vi "OAT Unfiltered Orbit Plot (Resampled).vi"(0 "resampled signal(X)":cluster{"r0":dbl, "dr":dbl, "Y":dbl[]} {"r0" format="%.2p"; "dr" format="%.2p"; "Y" format="%.2f"}, 1 "XY graph Ref":refnum<vi>, 5 "resampled signal (Y)":cluster{"r0":dbl, "dr":dbl, "Y":dbl[]} {"r0" format="%.2p"; "dr" format="%.2p"; "Y" format="%.2f"}, 7 "speed profile":T1 {"speed [RPM]" format="%.2f"; "time [s]" format="%.2f"}, 9 "pulse/revolution (1)":i32=1, 11 "error in (no error)":errorcluster, 12 "orbit segment":cluster{"position":dbl, "tach duty":dbl}={"position"=0.0, "tach duty"=0.98} {"tach duty" format="%.2f"; "position" format="%.2f"}, 13 "probe angle":u16(ring) items=["0", "45", "90", "135", "180", "225", "270", "315"]) -> (4 "XY plot value":cluster{"X":dbl[], "Y":dbl[]}[](array[cluster]) {"Y" format="%.2f"; "X" format="%.2f"}, 15 "error out":errorcluster)   [LabVIEW 2017]
doc: "Draws an orbit plot of waveform signals on a XY graph. You can use sampled or resampled waveform signals from proximity transducers. You can use this polymorphic VI to draw an orbit plot of resampled signals or waveform signals. The data types you wire to the <B>resampled signal(X)</B> and <B>resampled signal (Y)</B> inputs determine the polymorphic instance to use."
uses:
  <vilib>/addons/Sound and Vibration/Order Analysis/Tach Process/SubVIs/speed profile.ctl
  <vilib>/addons/Sound and Vibration/Order Analysis/Tach Process/SoundVib_TachProcess.lvlib
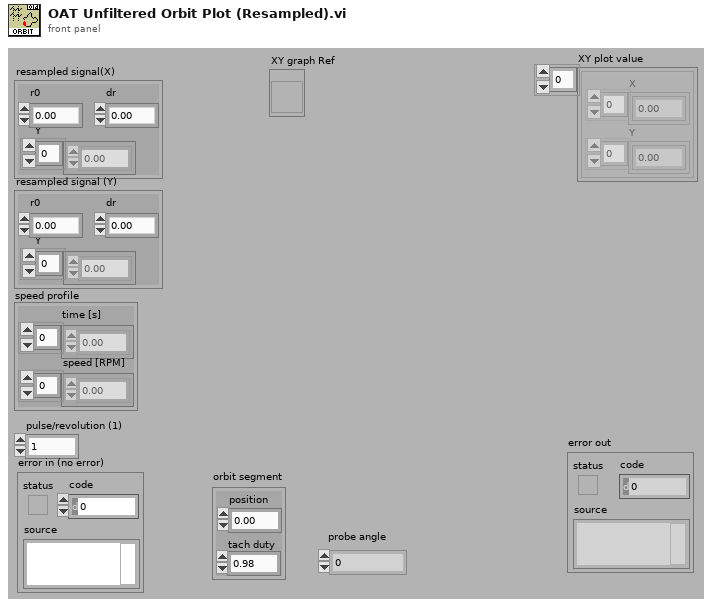
[diagram p1: front panel]
types:
  T1 = typedef "SoundVib_TachProcess.lvlib/speed profile.ctl" = cluster{"time [s]":dbl[], "speed [RPM]":dbl[]}
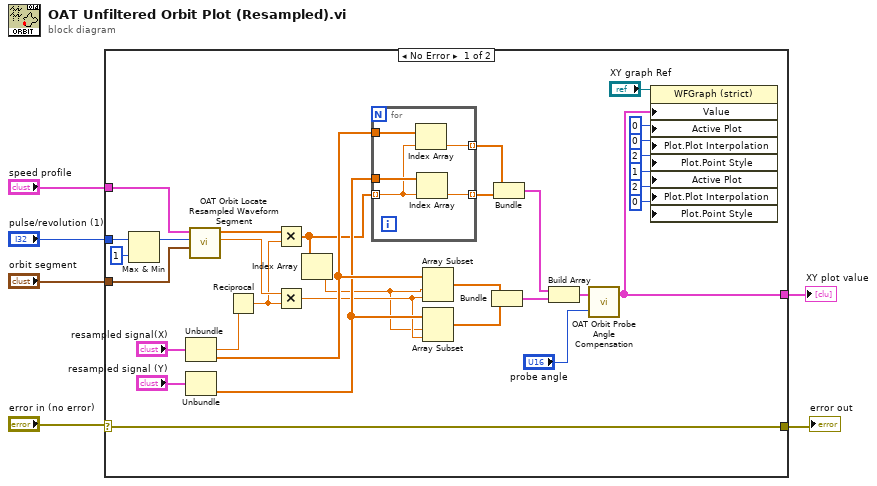
[diagram p0: block diagram]
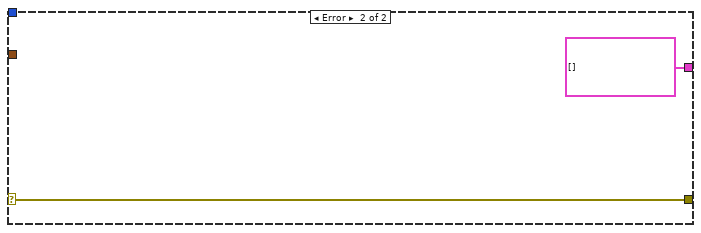
[diagram p2: hidden frame]
diagram:
  n1 = case shown="No Error" "error in (no error)" {
    selector: "error in (no error)" -> [w13 w46]
    tunnel: [w11 cluster{dbl[], dbl[]}[] []] -> w6
    tunnel: "speed profile" -> [w22 _]
    tunnel: "pulse/revolution (1)" -> [w9 _]
    tunnel: "orbit segment" -> [w21 _]
    tunnel: [w13 w46] -> w1
    frame No Error {
      n2 = Max & Min(x=w9, y=1) -> (max(x,y)=w8:i32)  [unwired: 1 out]
      n3 = Unbundle("resampled signal(X)") -> ("dr"=w20:dbl, "Y"=w25:dbl[])  [unwired: 1 out]
      n4 = Unbundle("resampled signal (Y)") -> ("Y"=w24:dbl[])  [unwired: 2 out]
      n5 = call <vilib>:"OAT Orbit Locate Resampled Waveform Segment.vi"("orbit segment"=w21, "pulse/revolution (1)"=w8, "speed profile"=w22) -> ("duration"=w18:dbl, "start points"=w19:dbl[])  [unwired: 6 in, 1 out]
      n6 = Reciprocal(x=w20) -> (1/x=w17:dbl)
      n7 = Multiply(x=w19, y=w17) -> (x*y=w15:dbl[])
      n8 = Multiply(x=w18, y=w17) -> (x*y=w16:dbl)
      n9 = Index Array(array=w15) -> (element=w14:dbl)  [unwired: 1 in]
      n10 = for {
        tunnel: [w44] -> w31 mode=indexing
        tunnel: [w42] -> w30 mode=indexing
        tunnel: w25 -> [w43]
        tunnel: w24 -> [w41]
        tunnel: w15 -> [w40] mode=indexing
        n11 = Index Array(array=w43, index=w40) -> (element=w44:dbl)
        n12 = Index Array(array=w41, index=w40) -> (element=w42:dbl)
      }
      n13 = Array Subset(array=w25, index=w14, length=w16) -> (w27:dbl[])
      n14 = Array Subset(array=w24, index=w14, length=w16) -> (w26:dbl[])
      n15 = Bundle(w27, w26) -> (w39:cluster{dbl[], dbl[]})  [unwired: 1 in]
      n16 = Bundle(w31, w30) -> (w23:cluster{dbl[], dbl[]})  [unwired: 1 in]
      n17 = Build Array(w23, w39) -> (w12:cluster{dbl[], dbl[]}[])
      n18 = call <vilib>:"OAT Orbit Probe Angle Compensation.vi"("probe angle compensation"="probe angle", "XY plot data in"=w12) -> ("XY plot data out"=w11:cluster{dbl[], dbl[]}[])  [unwired: 1 in]
      n19 = property class="WFGraph (strict)"(reference="XY graph Ref", "Value"=w11, "Active Plot"=u32 0, "Plot.Plot Interpolation"=u8 0, "Plot.Point Style"=u8 2, "Active Plot"=u32 1, "Plot.Plot Interpolation"=u8 2, "Plot.Point Style"=u8 0) -> ()  [unwired: 1 in, 2 out]
    }
    frame Error {
    }
  }
  "XY plot value" <- w6
  "error out" <- w1
